vi "Instrument Typecast.vi"(8 "error in (no error)":errorcluster, 11 "pin instrument":refnum<class>) -> (0 "error out":errorcluster, 3 "instrument object":refnum<class "Abstract_Instrument.lvclass">)   [LabVIEW 2021, in "Abstract_Instrument.lvclass"]
uses:
  Abstract_Instrument.lvclass
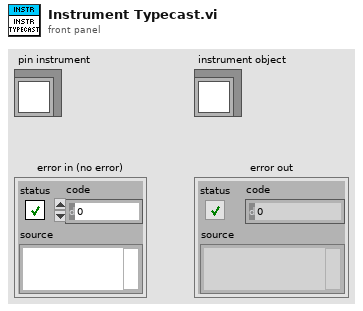
[diagram p1: front panel]
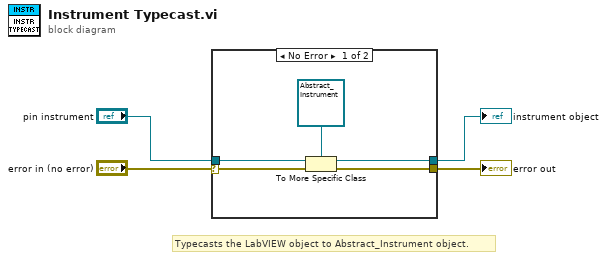
[diagram p0: block diagram]
diagram:
  # "Typecasts the LabVIEW object to Abstract_Instrument object."
  n1 = case shown="No Error" "error in (no error)" {
    selector: "error in (no error)" -> [w9 w10]
    tunnel: [w8 w10] -> w3
    tunnel: [w6 _] -> w2
    tunnel: "pin instrument" -> [w5 _]
    frame No Error {
      n2 = To More Specific Class(target class=refnum<class "Abstract_Instrument.lvclass"> refnum ("Abstract_Instrument.lvclass"), reference=w5, error in=w9) -> (specific class reference=w6:refnum<class "Abstract_Instrument.lvclass">, error out=w8:errorcluster)
    }
    frame Error {
    }
  }
  "error out" <- w3
  "instrument object" <- w2
